vi "Write Points.vi"(8 "error in (no error)":errorcluster, 10 "Points":T1[](array[typedef]), 11 "PathCommands in":refnum<class "PathCommands.lvclass">) -> (0 "error out":errorcluster, 3 "PathCommands out":refnum<class "PathCommands.lvclass">)   [LabVIEW 2019, in "PathCommands.lvclass"]
uses:
  PathCommands.lvclass
  Point.ctl
  PathCommands.lvclass/PathCommands.ctl
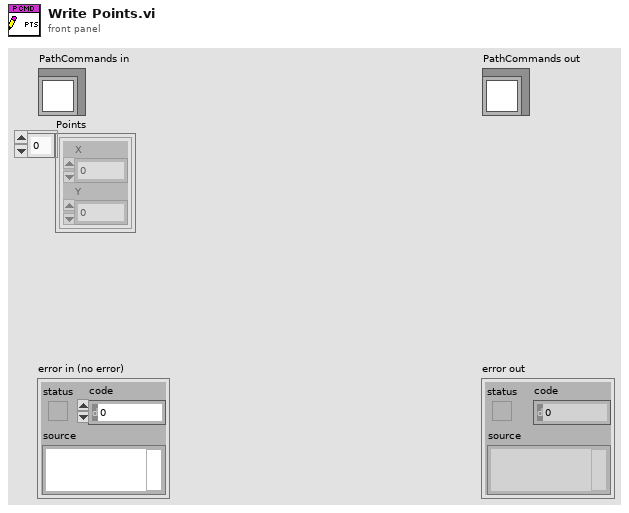
[diagram p1: front panel]
types:
  T1 = typedef "PathCommands.lvclass/Point.ctl" = cluster{"X":dbl, "Y":dbl}
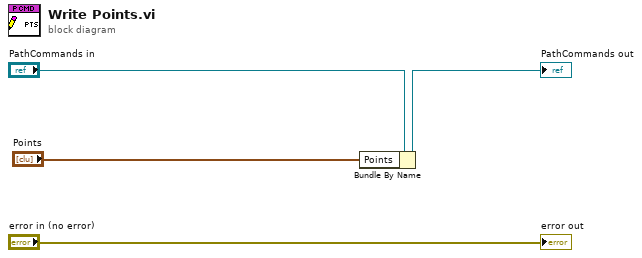
[diagram p0: block diagram]
diagram:
  n1 = Bundle By Name(cluster="PathCommands in", "Points"="Points") -> (→"PathCommands out":refnum<class "PathCommands.lvclass">)
  "error out" <- "error in (no error)"
